vi "test_leak2.vi"() -> ()   [LabVIEW 2020]
panel:
  out "error out":errorcluster
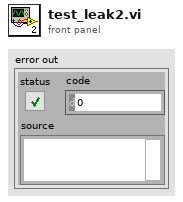
[diagram p1: front panel]
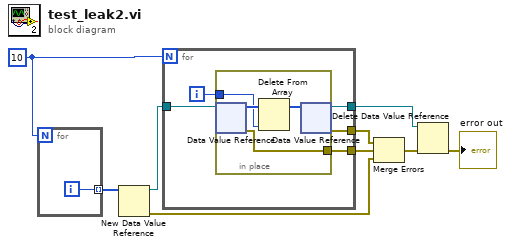
[diagram p0: block diagram]
diagram:
  w7 = 10
  n1 = for {
    N: w7 -> [_]
    tunnel: [w10] -> w9 mode=indexing
    i -> [w10]
  }
  n2 = New Data Value Reference(data value=w9) -> (data value reference=w8:refnum<data-value>, error out=w3:errorcluster)  [unwired: 1 in]
  n3 = for {
    N: w7 -> [_]
    tunnel: w8 -> [w15]
    tunnel: [w13] -> w6
    tunnel: [w12] -> w5
    tunnel: [w11] -> w4
    i -> [w14]
    n4 = in-place {
      in-place-border: w14 -> [w17]
      in-place-border: [w16] -> w11
      n5 = in-place-dvr #1(w15) -> (w19:i32[], w16:errorcluster)
      n6 = Delete From Array(array=w19, index=w17) -> (array with subset deleted=w18:i32[])  [unwired: 1 in, 1 out]
      n7 = in-place-dvr #1(w18) -> (w13:refnum<data-value>, w12:errorcluster)
    }
  }
  n8 = Merge Errors(w5, w4, w3) -> (w2:errorcluster)
  n9 = Delete Data Value Reference(data value reference=w6, error in=w2) -> (error out=→"error out":errorcluster)  [unwired: 1 out]
